vi "Error Bars.vi"() -> ()   [LabVIEW 2011]
uses:
  <vilib>/Heliosphere Research LLC/Advanced Plotting Toolkit/Advanced Plotting Toolkit.lvlib
  <vilib>/Heliosphere Research LLC/Advanced Plotting Toolkit/typedefs/PlotColor.ctl
  <vilib>/Heliosphere Research LLC/Advanced Plotting Toolkit/properties/Display.ctl
  <vilib>/Heliosphere Research LLC/Advanced Plotting Toolkit/api_plotting/ErrorbarProperties.ctl
panel:
  in  "Color":T1=2147483647 items=["Automatic"=2147483647, "Black"=0, "White"=16777215, "Red"=16711680, "Green"=2263842, "Blue"=255, "Cyan"=65535, "Magenta"=16711935, "Yellow"=16776960]
  in  "Cap Size":dbl=3.0
  in  "Line Width":dbl=1.0
  in  "Y Error Bars":bool=TRUE
  in  "X Error Bars":bool
  out "Errorbars":picture
  # "Error Bars"
  # "Error bars can be added to any 1D plot such as those made\nwith Line.vi, Scatter.vi, or Bar.vi.\n\nMake your plot first using the appropriate plotting VI.  Then\ncall Errorbar.vi to overlay the error bars.\n\nThe default color used for the bars is the last-used color in\nthe color cycle.  You can override this; try it below."
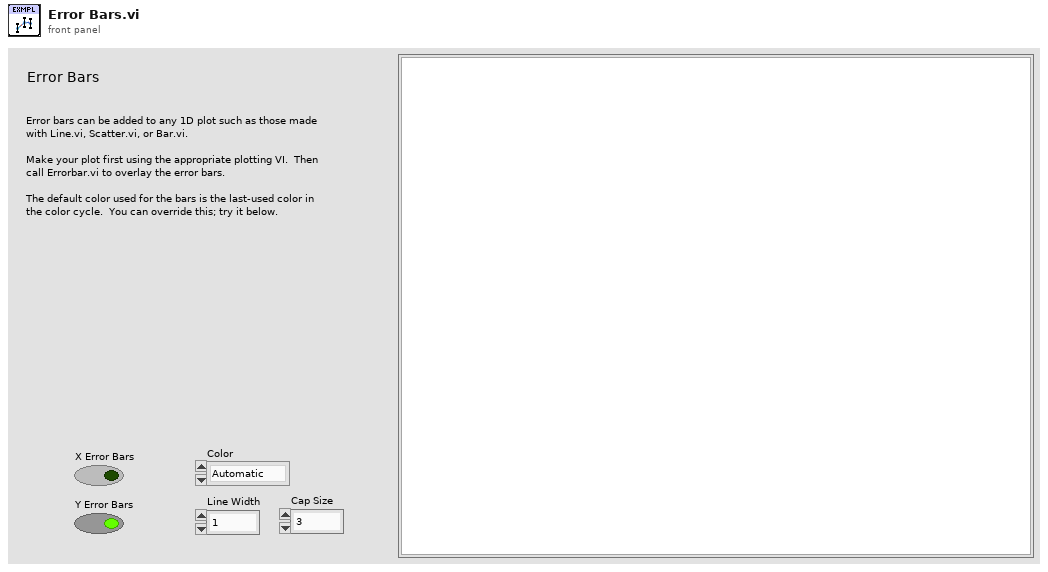
[diagram p1: front panel]
types:
  T1 = typedef "Advanced Plotting Toolkit.lvlib/PlotColor.ctl" = u32
  T2 = typedef "Advanced Plotting Toolkit.lvlib/ErrorbarProperties.ctl" = cluster{"Color":T1, "Line Width":dbl, "Cap Size":dbl, "Display":T3}
  T3 = typedef "Advanced Plotting Toolkit.lvlib/Display.ctl" = cluster{"Alpha":dbl, "Z Order":dbl}
  T4 = typedef "Advanced Plotting Toolkit.lvlib/PlotID.ctl" = i32
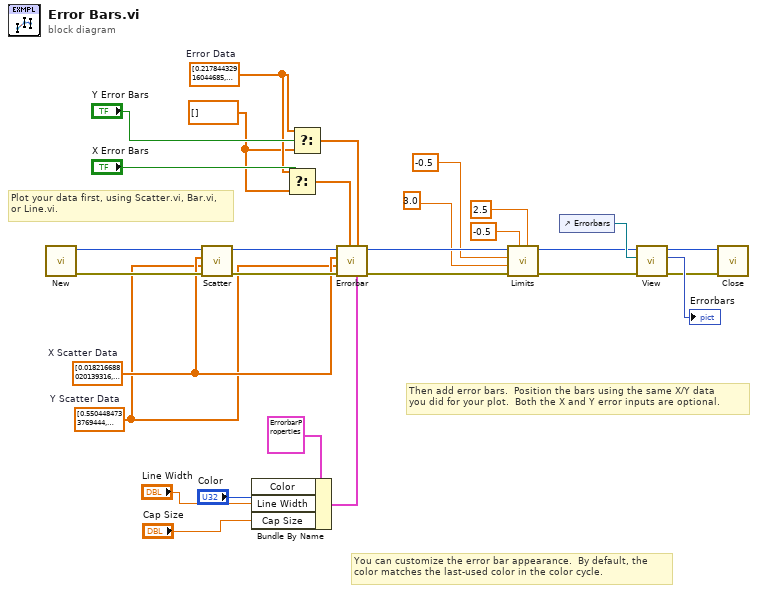
[diagram p0: block diagram]
diagram:
  w9 = dbl[] [] ("f")
  w17 = dbl[] [0.21784432916044685, 0.30622571626809264, 0.23973331815755852, 0.27715181252061744, 0.2897801865085579, 0.19272493092782117, 0.2523775836791941, 0.27705982683566244, 0.2622653367158178, 0.31348737463659937, 0.26239385585263925, 0.20942940502020338, 0.30280631894863735, 0.21505853526341212, 0.28472832872399834, 0.24113153620062713, 0.2073508820740427, 0.19647038643673007, 0.21482885996797138, 0.3030383238021465, 0.19907177450068972, 0.22230733575951378, 0.3100041798921069, 0.29007788384152905, 0.19437691444769178, 0.3028584951872156, 0.25704184950497794, 0.19020235317422807, 0.27229412146187254, 0.2852580302988544, 0.19307859892266951, 0.3101282589800766, 0.2500909796828448, 0.27662896478236243, 0.296436603677368, 0.1946491263789194, 0.2323244497194478, 0.21429614824029017, 0.2197387433660547, 0.2808346398127908, 0.2925053806173366, 0.18536660722012158, 0.20185386963566673, 0.2581518005352822, 0.1908197246675424, 0.22060531735843225, 0.2447222843938961, 0.19234260957244467, 0.22119863157479247, 0.17402860686679644]  # Error Data
  w21 = dbl[] [0.5504484733769444, 0.7340145289331643, 0.9972841843730318, 0.739103164755676, 0.4719489274133991, 0.48521359909880923, 0.268670749089941, 0.8057782296946243, 0.9028181748401577, 0.7301380893918062, 0.5945088382745651, 0.5664841888262767, 0.6245603532933975, 1.2151753773851341, 1.3751559325201912, 0.7594195233427825, 0.9174437047884547, 0.888032137496148, 1.027309928555396, 0.8465183772390145, 1.4611410254800308, 0.7854320310413877, 1.3305249271114152, 1.4337017682881403, 0.8238392444886502, 1.4695688108297478, 1.5221063546175306, 0.8713493416820589, 1.0954736948939998, 1.6983962844027416, 1.3662143684153685, 1.2125284144057185, 1.1981155398847738, 1.6763550413556394, 1.521911612001944, 1.3177646228410758, 1.413803334048454, 1.639339701921609, 1.6199879794898349, 1.68887714231835, 1.561633324060962, 1.9041851472536078, 1.3852047085256352, 1.7361658644546871, 1.699321108236791, 1.9305833477615097, 1.5819086670974714, 1.7707421705426076, 1.6307798240979468, 1.7271994646006077]  # Y Scatter Data
  w22 = dbl[] [0.018216688020139316, 0.6155646664152035, 0.09161887446563804, 0.5755835424122354, 0.30811405678216486, 0.9300868119887228, 0.7586483780489142, 1.089769759555441, 0.6322835384289796, 0.384787183193845, 1.2778344980742953, 0.9812998154301975, 0.3864217942054192, 1.2257226583790302, 0.5022360656236784, 1.4019622035534751, 0.6452632674815559, 0.8791971175839632, 0.8100268209069452, 1.3321489027970501, 0.6454080555060299, 1.6038888739516306, 0.9794885993611202, 1.201703057246671, 1.3700683222399341, 1.3958110923468907, 1.5420824872003653, 1.5316056401142393, 0.9179293358604258, 1.0770885097208276, 1.0840019398416834, 1.9012209722097482, 1.0103364765183542, 1.4257742799494155, 1.6657001005581127, 1.6988166953387351, 1.6494618253350257, 2.0765624770416053, 2.0856701722269166, 1.4103354500274605, 1.4609448842344637, 2.0763197759765175, 1.6784655640635633, 1.9584138400305964, 2.312762778270861, 1.5973704682789003, 2.0813213329442646, 1.9574908741379595, 2.229063128359036, 1.9824983595019636]  # X Scatter Data
  # "You can customize the error bar appearance.  By default, the\ncolor matches the last-used color in the color cycle."
  # "Then add error bars.  Position the bars using the same X/Y data\nyou did for your plot.  Both the X and Y error inputs are optional."
  # "Plot your data first, using Scatter.vi, Bar.vi,\nor Line.vi."
  n1 = call <vilib>:"New.vi"() -> ("error out"=w25:errorcluster, "Plot ID"=w26:T4)  [unwired: 10 in]
  n2 = call <vilib>:"Scatter.vi"("error in (no error)"=w25, "Y Data"=w21, "X Data"=w22, "Plot ID"=w26) -> ("error out"=w23:errorcluster, "Plot ID Out"=w24:T4)  [unwired: 6 in]
  n3 = Bundle By Name(cluster=T2 {"Color"=2147483647, "Line Width"=nan, "Cap Size"=nan, "Display"={"Alpha"=nan, "Z Order"=nan}} ("Errorbar Properties"), "Color"="Color", "Line Width"="Line Width", "Cap Size"="Cap Size") -> (w5:T2)
  n4 = Select(t=w17, s="X Error Bars", f=w9) -> (s? t:f=w19:dbl[])
  n5 = Select(t=w17, s="Y Error Bars", f=w9) -> (s? t:f=w16:dbl[])
  n6 = call <vilib>:"Errorbar.vi"("Properties"=w5, "Y Errors"=w16, "X Errors"=w19, "error in (no error)"=w23, "Y Data"=w21, "X Data"=w22, "Plot ID"=w24) -> ("error out"=w14:errorcluster, "Plot ID out"=w15:T4)  [unwired: 3 in]
  n7 = call <vilib>:"Limits.vi"("Y Max"=2.5, "Y Min"=-0.5, "error in (no error)"=w14, "X Max"=3.0, "X Min"=-0.5, "Plot ID"=w15) -> ("error out"=w2:errorcluster, "Plot ID Out"=w3:T4)  [unwired: 4 in]
  n8 = control-ref of="Errorbars"() -> (w29:refnum<vi>)
  n9 = call <vilib>:"View.vi"("error in (no error)"=w2, "Ref for Sizing"=w29, "Plot ID"=w3) -> ("error out"=w1:errorcluster, "Picture"=→"Errorbars":picture, "Plot ID Out"=w27:T4)  [unwired: 6 in]
  n10 = call <vilib>:"Close.vi"("error in (no error)"=w1, "Plot ID"=w27) -> ()  [unwired: 9 in, 1 out]
